vi "Colormaps2004.vi"   [LabVIEW 2013]
uses:
  <vilib>/Heliosphere Research LLC/Advanced Plotting Toolkit/api_plotting/ArrayViewProperties.ctl
  <vilib>/Heliosphere Research LLC/Advanced Plotting Toolkit/properties/Colormap.ctl
  <vilib>/Heliosphere Research LLC/Advanced Plotting Toolkit/properties/Colormap_Map.ctl
  <vilib>/Heliosphere Research LLC/Advanced Plotting Toolkit/properties/Colormap_Scaling.ctl
  <vilib>/Heliosphere Research LLC/Advanced Plotting Toolkit/properties/Display.ctl
  <vilib>/Heliosphere Research LLC/Advanced Plotting Toolkit/Advanced Plotting Toolkit.lvlib
types:
  T1 = typedef "Advanced Plotting Toolkit.lvlib/Colormap_Map.ctl" = enum16{"Automatic", "Rainbow", "Hot and Cold", "White-Black", "White-Blue", "White-Green", "White-Red", "Fire", "Water", "Earth", "Air", "Pastel", "Banded", "Stepped"}
  T2 = typedef "Advanced Plotting Toolkit.lvlib/ArrayViewProperties.ctl" = cluster{"Colormap":T3, "Display":T5}
  T3 = typedef "Advanced Plotting Toolkit.lvlib/Colormap.ctl" = cluster{"Map":T1, "Value Min":dbl, "Value Max":dbl, "Scaling":T4, "Reverse":bool}
  T4 = typedef "Advanced Plotting Toolkit.lvlib/Colormap_Scaling.ctl" = enum16{"Default"}
  T5 = typedef "Advanced Plotting Toolkit.lvlib/Display.ctl" = cluster{"Alpha":dbl, "Z Order":dbl}
  T6 = typedef "Advanced Plotting Toolkit.lvlib/PlotID.ctl" = i32
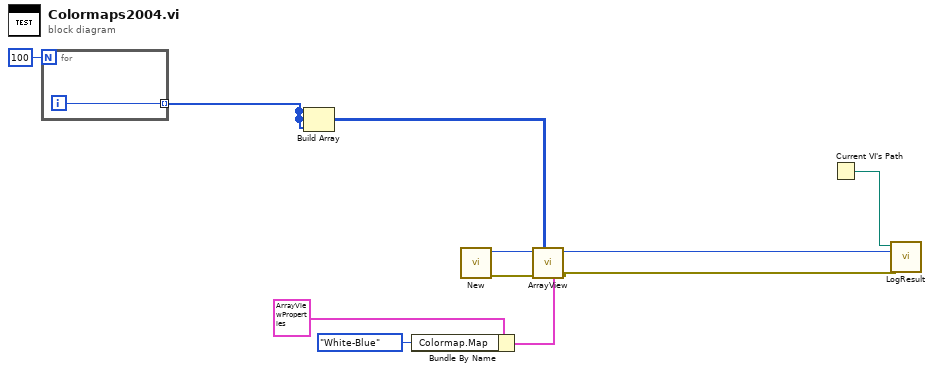
[diagram p0: block diagram]
diagram:
  n1 = for {
    N: 100 -> [_]
    tunnel: [w12] -> w3 mode=indexing
    i -> [w12]
  }
  n2 = Build Array(w3, w3, w3) -> (w1:i32[][])
  n3 = Bundle By Name(cluster=T2 {"Colormap"={"Map"=enum."Automatic", "Value Min"=nan, "Value Max"=nan, "Scaling"=enum."Default", "Reverse"=FALSE}, "Display"={"Alpha"=nan, "Z Order"=nan}} ("Array View Properties"), "Colormap.Map"=Colormap_Map."White-Blue") -> (w5:T2)
  n4 = call <vilib>:"New.vi"() -> ("error out"=w8:errorcluster, "Plot ID"=w9:T6)  [unwired: 10 in]
  n5 = call <vilib>:"ArrayView.vi"("Properties"=w5, "Data"=w1, "error in (no error)"=w8, "Plot ID"=w9) -> ("error out"=w7:errorcluster, "Plot ID Out"=w10:T6)  [unwired: 6 in]
  n6 = Current VI's Path() -> (path=w11:path)
  n7 = call "LogResult.vi"("Test Result"=w7, "Test Artifact"=w10, "VI Path"=w11) -> ()  [unwired: 9 in]
